vi "Append Loaded Sequences.vi"(8 "error in (no error)":errorcluster, 10 "Array of Seqs Loaded":refnum<class "Sequence of SBlocks.lvclass">[](array[class]), 11 "Scheduler in":refnum<class "Scheduler.lvclass">) -> (0 "error out":errorcluster, 3 "Scheduler out":refnum<class "Scheduler.lvclass">)   [LabVIEW 2020, in "Scheduler.lvlib" / "Scheduler.lvclass"]
uses:
  Scheduler.lvclass
  Run Utilities/Sequence of SBlocks/Sequence of SBlocks.lvclass
  Scheduler.lvclass/Scheduler.ctl
  Ancestor/Ancestor/Ancestor.lvclass/Ancestor.ctl
  86217c6a-0f82-465d-b7e1-daf06c0e6fb5.vi
  Support VIs/Generate Error.vi
  FGV/Error Memory/Get Error Description.vi
  Support VIs/Get PC name.vi
  Ancestor/Ancestor/Read ID.vi
  Support VIs/Get Class Name.vi
  <vilib>/Utility/error.llb/Clear Errors.vi
  FGV/Error Memory/Error Memory Core.vi
  <vilib>/AdvancedString/Delimited String to 1D String Array.vi
  Support VIs/Circus Root Path.vi
  FGV/Error Memory/Error Crt Lvl checker.vi
  FGV/Error Memory/Error Memory Core.vi/40c8088d-b597-4017-91af-faa98e00292e.vi
  FGV/Error Memory/Error Memory Core.vi/d4a3ab98-063c-4e44-b43d-fbdcfe6c2be2.vi
  Support VIs/Global Memory.vi
  <vilib>/Utility/LVClass/Get LV Class Name.vi
  Support VIs/Is in Packed Library.vi
  Support VIs/TALOS Root path.vi
  Support VIs/Read CSV worksheet.vi
  Support VIs/Global Constants.vi
  <vilib>/Utility/error.llb/General Error Handler.vi
  Support VIs/Error Log.vi
  <vilib>/Comparison/Equal/Equal Functor/Equal Functor.lvclass
  Ancestor/Ancestor/Ancestor.lvclass
  TALOS.lvlib
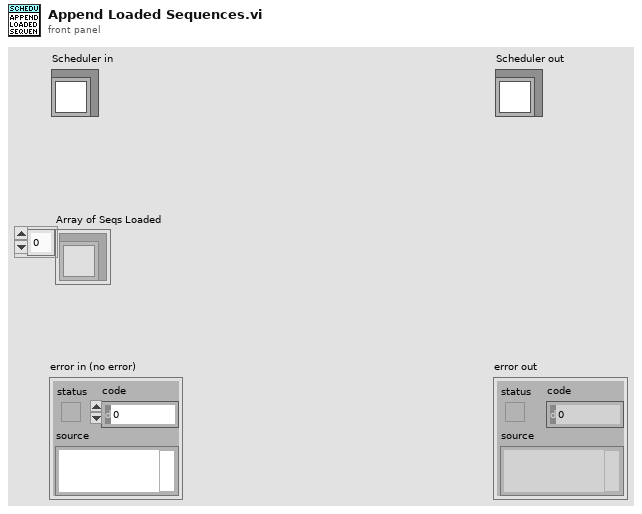
[diagram p1: front panel]
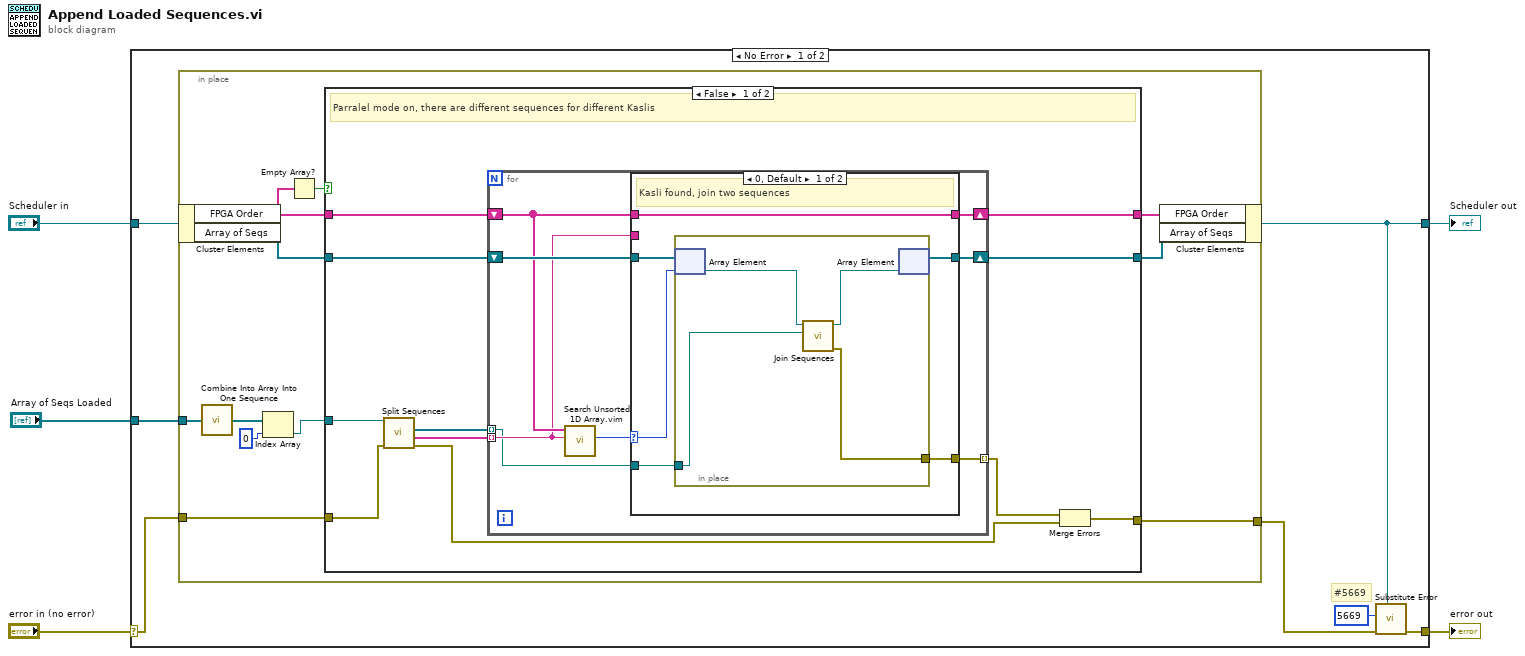
[diagram p0: block diagram]
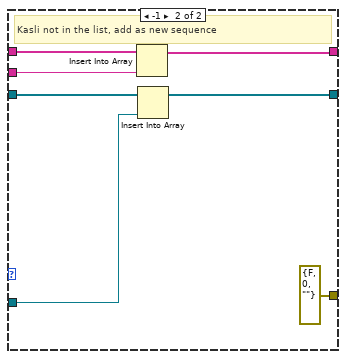
[diagram p2: hidden frame]
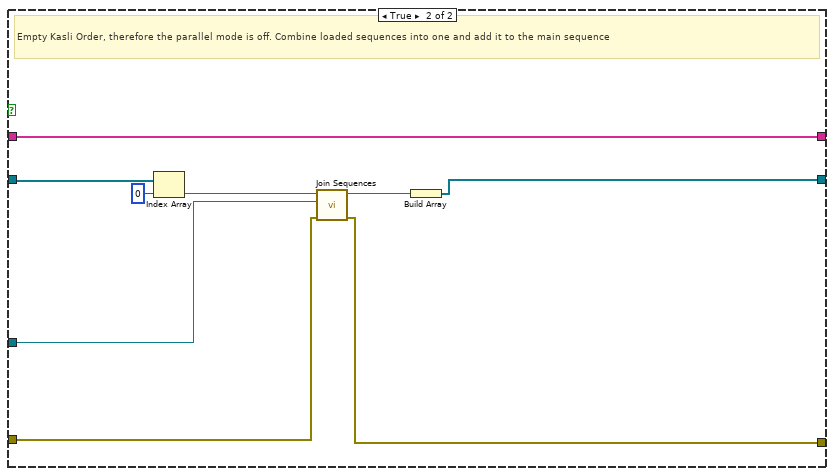
[diagram p3: hidden frame]
diagram:
  n1 = case shown="No Error" "error in (no error)" {
    selector: "error in (no error)" -> [w10 w70]
    tunnel: [w9 w70] -> w4
    tunnel: [w7 w69] -> w2
    tunnel: "Scheduler in" -> [w12 w69]
    tunnel: "Array of Seqs Loaded" -> [w11 _]
    frame No Error {
      # "#5669"
      n2 = in-place {
        in-place-border: w11 -> [w18]
        in-place-border: w10 -> [w14]
        in-place-border: [w13] -> w8
        n3 = in-place-cluster #1(w12) -> ("FPGA Order"=w22:string[], "Array of Seqs"=w20:refnum<class "Sequence of SBlocks.lvclass">[])
        n4 = call "Combine Into Array Into One Sequence.vi"("Array of Seqs in"=w18) -> ("Array of Seqs out"=w17:refnum<class "Sequence of SBlocks.lvclass">[])
        n5 = Index Array(array=w17, index=0) -> (element=w15:refnum<class "Sequence of SBlocks.lvclass">)
        n6 = Empty Array?(array=w22) -> (empty?=w23:bool)
        n7 = case shown="False" w23 {
          tunnel: w20 -> [w31 w68]
          tunnel: [w29 w65] -> w19
          tunnel: w22 -> [w32 w64]
          tunnel: [w28 w64] -> w21
          tunnel: w15 -> [w34 w63]
          tunnel: w14 -> [w27 w61]
          tunnel: [w24 w60] -> w13
          frame False {
            # "Parralel mode on, there are different sequences for different Kaslis"
            n8 = call "Split Sequences.vi"("error in (no error)"=w27, "Sequence of SBlocks in"=w34) -> ("error out"=w25:errorcluster, "Kasli Order"=w33:string[], "Array of Sequences"=w30:refnum<class "Sequence of SBlocks.lvclass">[])  [unwired: 6 in, 1 out]
            n9 = for {
              tunnel: w33 -> [w37] mode=indexing
              shift-right: [w38] -> w28
              shift-left: w32 -> [w39]
              shift-right: [w40] -> w29
              shift-left: w31 -> [w41]
              tunnel: w30 -> [w36] mode=indexing
              tunnel: [w35] -> w26 mode=indexing
              n10 = call "Search Unsorted 1D Array.vim"("element"=w37, "unsorted 1D array"=w39) -> ("index of element"=w42:i32)  [unwired: 9 in]
              n11 = case shown="0, Default" w42 {
                selector: w42 -> [w46 _]
                tunnel: w41 -> [w47 w59]
                tunnel: [w44 w58] -> w40
                tunnel: w39 -> [w48 w57]
                tunnel: [w48 w56] -> w38
                tunnel: w37 -> [_ w55]
                tunnel: w36 -> [w45 w54]
                tunnel: [w43 errorcluster {"status"=FALSE, "code"=0, "source"=""} ("error out")] -> w35
                frame 0, Default {
                  # "Kasli found, join two sequences"
                  n12 = in-place {
                    in-place-border: w45 -> [w52]
                    in-place-border: [w49] -> w43
                    n13 = in-place-array #2(w47, w46) -> (w51:refnum<class "Sequence of SBlocks.lvclass">)
                    n14 = call-dynamic "Join Sequences.vi"("Sequence of SBlocks"=w52, "Sequence of SBlocks in"=w51) -> ("error out"=w49:errorcluster, "Sequence of SBlocks out"=w50:refnum<class "Sequence of SBlocks.lvclass">)  [unwired: 8 in]
                    n15 = in-place-array #2(w50) -> (w44:refnum<class "Sequence of SBlocks.lvclass">[])  [unwired: 1 out]
                  }
                }
                frame -1 {
                  # "Kasli not in the list, add as new sequence"
                  n16 = Insert Into Array(array=w57, new element=w55) -> (w56:string[])  [unwired: 1 in]
                  n17 = Insert Into Array(array=w59, new element=w54) -> (w58:refnum<class "Sequence of SBlocks.lvclass">[])  [unwired: 1 in]
                }
              }
            }
            n18 = Merge Errors(w26, w25) -> (w24:errorcluster)
          }
          frame True {
            # "Empty Kasli Order, therefore the parallel mode is off. Combine loaded sequences into one and add it to the main sequence"
            n19 = Index Array(array=w68, index=0) -> (element=w67:refnum<class "Sequence of SBlocks.lvclass">)
            n20 = call-dynamic "Join Sequences.vi"("error in (no error)"=w61, "Sequence of SBlocks"=w63, "Sequence of SBlocks in"=w67) -> ("error out"=w60:errorcluster, "Sequence of SBlocks out"=w66:refnum<class "Sequence of SBlocks.lvclass">)  [unwired: 7 in]
            n21 = Build Array(w66) -> (w65:refnum<class "Sequence of SBlocks.lvclass">[])
          }
        }
        n22 = in-place-cluster #1("FPGA Order"=w21, "Array of Seqs"=w19) -> (w7:refnum<class "Scheduler.lvclass">)
      }
      n23 = call "Substitute Error.vi"("LabVIEW Object"=w7, "error in (no error)"=w8, "Error Code"=5669) -> ("error out"=w9:errorcluster)  [unwired: 8 in]
    }
    frame Error {
    }
  }
  "error out" <- w4
  "Scheduler out" <- w2
